vi "Row_Col_Dot_withshift.vi"(6 "Shift":u16=9, 8 "NS":u16=9, 10 "X":sgl[](array[numeric])=[1.0, 2.0, 3.0, 4.0, 5.0, 6.0, 7.0, 8.0, 9.0, 0.0, 0.0, 0.0, 0.0, 0.0, 0.0, 0.0, 0.0, 0.0, 0.0, 0.0, 0.0, 0.0, 0.0, 0.0, 0.0], 11 "Refnum in":refnum<k21>="AasCol 2") -> (2 "a^t*x":sgl format="%#_13g")   [LabVIEW 2017]
doc: "Given an input array X and a reference to a memory item, comput the dot product,\neg K.*X. X can be a vector up to length = 9.\n\nND is the size of the vectors.\n\n\nTHIS VI IS DIFFERENT FROM \"SGL_K2_times_xd\" by different sizes allowed."
uses:
  <vilib>/Platform/TimedLoop/XDataNode/timing_clust.ctl
  <vilib>/Platform/TimedLoop/XDataNode/nitl_modes.ctl
  <vilib>/Platform/TimedLoop/XDataNode/wakeup.ctl
  <vilib>/rvi/Emulation/niFpgaSctlEmulationGetInTimedLoop.vi
  <vilib>/rvi/Emulation/niFpgaEmulationReportErrorSimple.vi
  <vilib>/rvi/Emulation/niFpgaGetClockAttributes.vi
  <vilib>/rvi/Emulation/niFpgaCriticalErrorInLSC.vi
  <vilib>/rvi/DataTransferAndStorage/Container/Common/niFpgaContainerExecOnDevCompGetState.vi
  <vilib>/rvi/Emulation/niFpgaEmulationIsFPGAContextNoSignature.vi
  <vilib>/rvi/DataTransferAndStorage/Container/Common/niFpgaContainerGetUniqueNameForEmu.vi
  <vilib>/rvi/Emulation/niFpgaProcessEmulError.vi
  <vilib>/rvi/errors/nirviReportUnexpectedCaseInternalError (U32).vi
  <vilib>/rvi/Memory/Memory_Emulation/niFpgaMemoryEmulationCacheClearOnFirstRun.vi
  <vilib>/rvi/Memory/Memory_Emulation/nirvimemoryEmulationManagerCache_MakeExclusive.vi
  <vilib>/rvi/Memory/Memory_Emulation/niFpgaMemoryEmulationValidateCache.vi
  <vilib>/rvi/Memory/Memory_Emulation/nirvimemoryEmulationManagerCache_InsertValue.vi
  <vilib>/Utility/error.llb/Clear Errors.vi
  <vilib>/rvi/Memory/Memory_Emulation/nirvimemoryEmulationManagerCache_ReleaseExclusive.vi
  <vilib>/rvi/Memory/Memory_Emulation/nirvimemoryEmulationManagerCache_GetValue.vi
  <vilib>/rvi/Memory/Memory_Emulation/nirvimemoryEmulationManagerCache_SetValue.vi
  <vilib>/rvi/Emulation/niFpgaSctlEmulationResourceMgr.vi
  <vilib>/Platform/TimedLoop/XDataNode/XDataNode.xnode
  <vilib>/rvi/DataTransferAndStorage/Container/XNode/niFpgaContainer.xnode
  <vilib>/rvi/Memory/Memory_Emulation/niFpgaMemoryEmulationRefIn.vi
  <vilib>/Platform/TimedLoop/XDataNode/XDNodeRunTimeDep.lvlib
panel:
  # "This VI performs the dot product between a memory item (row vector)\nand a column vector in an array. The beginning position in the memory item\nis determined by the \"shift\" variable. This is useful in moving through a rectuangular\nmatrix stored as a column, all in one memory item."
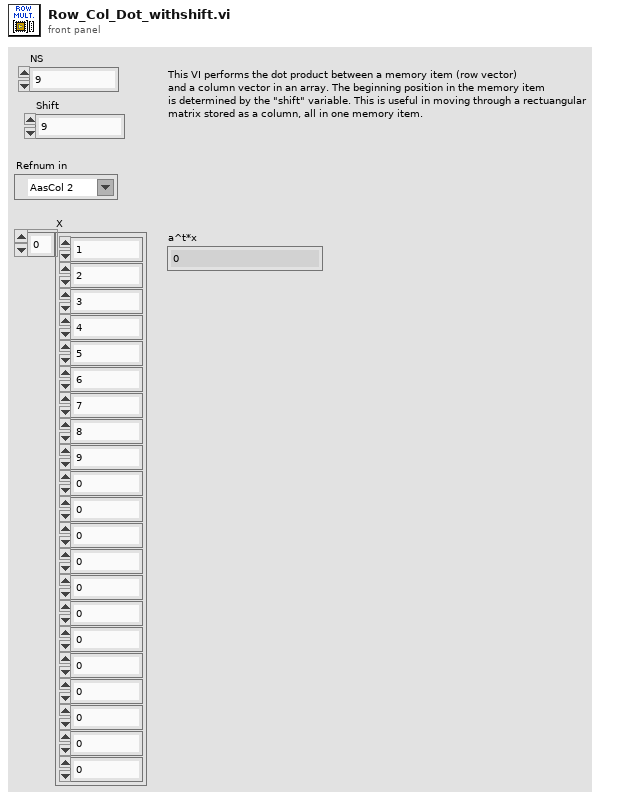
[diagram p1: front panel]
types:
  T1 = typedef "XDNodeRunTimeDep.lvlib/timing_clust.ctl" = cluster{"Expected End [f-1]":u64, "Actual End [f-1]":u64, "Finished Late? [f-1]":bool, "Expected End [i-1]":u64, "Actual End [i-1]":u64, "Finished Late? [i-1]":bool, "Expected Start [i]":u64, "Actual Start [i]":u64, "Expected Start [f]":u64, "Actual Start [f]":u64, "Source Name":string, "Structure Name":string, "Period":i64, "Deadline":i64, "Offset":i64, "Start":i64, "Priority":i32, "Timeout":i32, "Mode":T2, "Wakeup Reason":T3, "Error":errorcluster, "Source Type":string, "Secondary Source Type":string, "Global End Time":u64, "Global Start Time":u64, "Frame Duration":u64, "Iteration Duration":u64, "Assigned CPU":i32, "I/O Scan Engine Mode":u32}
  T2 = typedef "XDNodeRunTimeDep.lvlib/nitl_modes.ctl" = enum32{"No Change", "Process missed periods, maintain original phase", "Discard missed periods, maintain original phase", "Process missed periods, ignore original phase", "Discard missed periods, ignore original phase"}
  T3 = typedef "XDNodeRunTimeDep.lvlib/wakeup.ctl" = enum32{"Normal", "Aborted", "Asynchronous wakeup", "Timing source error", "Timed loop error", "Timeout"}
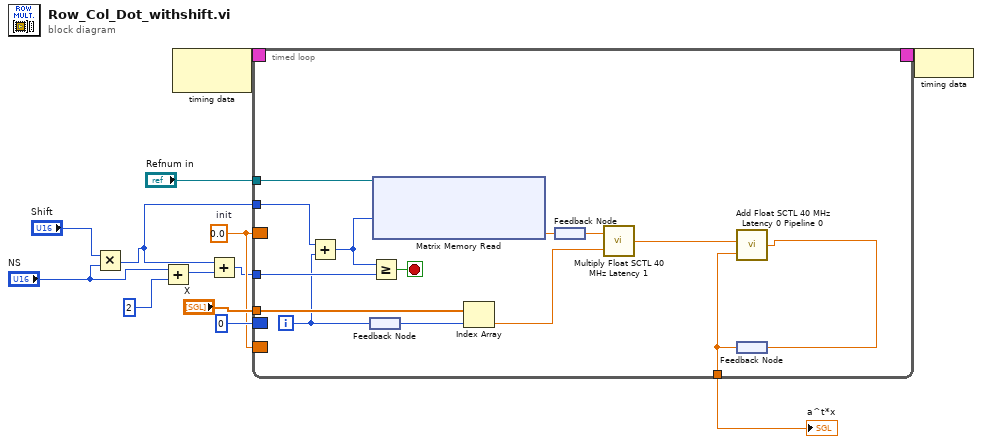
[diagram p0: block diagram]
diagram:
  w8 = sgl 0.0  # init
  n1 = Multiply(x="Shift", y="NS") -> (x*y=w4:u16)
  n2 = Add(x="NS", y=2) -> (x+y=w6:i32)
  n3 = node-c288() -> (w13:T1)  [unwired: 1 in]
  n4 = Add(x=w4, y=w6) -> (x+y=w5:i32)
  n5 = timed-loop {
    timing: w13 -> [_]
    timing-out: [_] -> w12
    border: w8 -> [_]
    tunnel: "Refnum in" -> [w26]
    tunnel: "X" -> [w25]
    border: 0 -> [_]
    tunnel: w5 -> [w23]
    border: w8 -> [_]
    tunnel: w4 -> [w19]
    tunnel: [w15] -> w3
    i -> [w20]
    stop <- w27 stop-if-true
    n6 = Add(x=w19, y=w20) -> (x+y=w18:i32)
    n7 = feedback #1() -> (w24:i32)
    n8 = feedback-in #1(w20) -> ()
    n9 = Greater Or Equal?(x=w18, y=w23) -> (x >= y?=w27:bool)
    n10 = xnode "Matrix Memory Read"("Address"=w18, "Memory In"=w26) -> ("Data"=w14:sgl)  [unwired: 1 out]
    n11 = Index Array(array=w25, index=w24) -> (element=w16:sgl)
    n12 = feedback #2() -> (w17:sgl)
    n13 = feedback-in #2(w14) -> ()
    n14 = call "Multiply Float SCTL 40 MHz Latency 1.vi"("y"=w16, "x"=w17) -> ("x[k-1]*y[k-1]"=w21:sgl)
    n15 = feedback #3() -> (w15:sgl)
    n16 = call "Add Float SCTL 40 MHz Latency 0 Pipeline 0.vi"("y"=w15, "x"=w21) -> ("x+y"=w22:sgl)
    n17 = feedback-in #3(w22) -> ()
  }
  "a^t*x" <- w3
  n18 = node-c288(w12) -> ()
